vi "Write DiffIO Setup.vi"(8 "error in (no error)":errorcluster, 10 "DiffIO Setup":T1[](array[typedef]) {"Skip Fire Index" max=7; "Angles"."Duration [s]" format="%#_3p"; "Frequency [Hz]" format="%#_3p"}, 11 "DCM-DSI-HW in":refnum<class "DCM-DSI.lvclass">) -> (0 "error out":errorcluster, 3 "DCM-DSI-HW out":refnum<class "DCM-DSI.lvclass">)   [LabVIEW 2016, in "DCM-DSI.lvclass"]
uses:
  DCM-DSI.lvclass
  <vilib>/Powertrain Controls/Device Drivers/DCM/Diff IO/RT/Setup.ctl
  <vilib>/Powertrain Controls/Device Drivers/DCM/Diff IO/FPGA/Mode.ctl
  <vilib>/Powertrain Controls/Device Drivers/DCM/Diff IO/RT/Angle Control.ctl
  DCM-DSI.lvclass/DCM-DSI.ctl
  <vilib>/Powertrain Controls/Device Drivers/DCM/Diff IO/FPGA/DCM - FPGA - Diff IO.lvlib
  <vilib>/Powertrain Controls/Device Drivers/DCM/Diff IO/RT/DCM - RT - Diff IO.lvlib
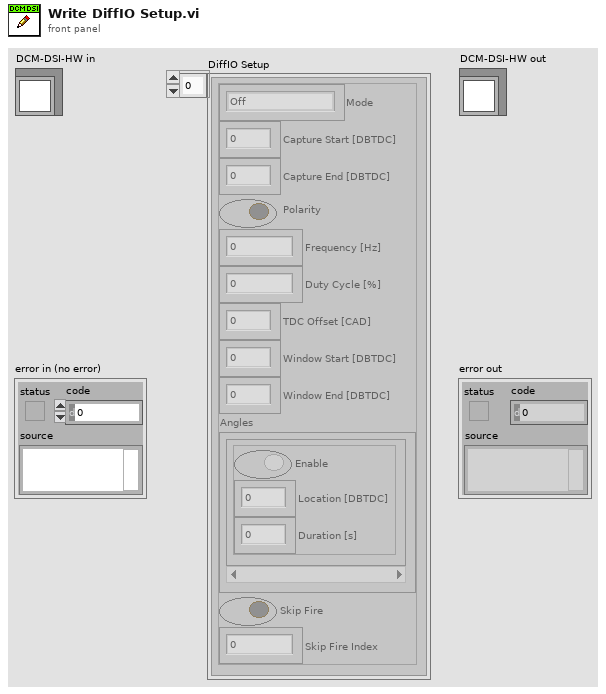
[diagram p1: front panel]
types:
  T1 = typedef "DCM - RT - Diff IO.lvlib/Setup.ctl" = cluster{"Mode":T2, "Capture Start [DBTDC]":sgl, "Capture End [DBTDC]":sgl, "Polarity":bool, "Frequency [Hz]":sgl, "Duty Cycle [%]":sgl, "TDC Offset [CAD]":sgl, "Window Start [DBTDC]":sgl, "Window End [DBTDC]":sgl, "Angles":T3[], "Skip Fire":bool, "Skip Fire Index":u8}
  T2 = typedef "DCM - FPGA - Diff IO.lvlib/Mode.ctl" = enum8{"Off", "Input", "Pulse Width Modulation", "Engine Position Tracking", "Serial Out 1", "Serial Out 2"}
  T3 = typedef "DCM - RT - Diff IO.lvlib/Angle Control.ctl" = cluster{"Enable":bool, "Location [DBTDC]":sgl, "Duration [s]":sgl}
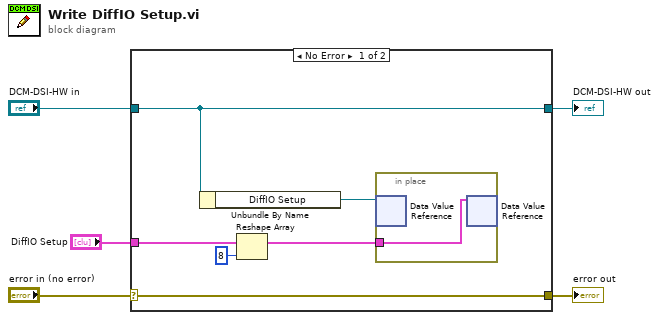
[diagram p0: block diagram]
diagram:
  n1 = case shown="No Error" "error in (no error)" {
    selector: "error in (no error)" -> [w11 w14]
    tunnel: [w11 w14] -> w4
    tunnel: [w9 w13] -> w2
    tunnel: "DCM-DSI-HW in" -> [w9 w13]
    tunnel: "DiffIO Setup" -> [w8 _]
    frame No Error {
      n2 = Unbundle By Name(w9) -> ("DiffIO Setup"=w10:refnum<data-value>)
      n3 = Reshape Array(w8, 8 ("dimension size")) -> (w7:T1[])
      n4 = in-place {
        in-place-border: w7 -> [w12]
        n5 = in-place-dvr #1(w10) -> ()  [unwired: 2 out]
        n6 = in-place-dvr #1(w12) -> ()  [unwired: 2 out]
      }
    }
    frame Error {
    }
  }
  "error out" <- w4
  "DCM-DSI-HW out" <- w2
